vi "DB_LeeIDmedicion.vi"(8 "error in (no error)":errorcluster, 10 "Equipo_Medicion in":T1={"ID_EQUIPO"=0, "IP_EQUIPO"="", "NOMBRE_EQUIPO"="", "ESTADO_EQUIPO"="", "DESCRIPCION"="", "ID_MEDICION"=0, "ESTADO_MEDICION"="", "TIEMPO_MEDICION"="12-02-2019 18:41"}, 11 "db in":T2) -> (0 "error out":errorcluster, 2 "Equipo_Medicion out":T1={"ID_EQUIPO"=0, "IP_EQUIPO"="", "NOMBRE_EQUIPO"="", "ESTADO_EQUIPO"="", "DESCRIPCION"="", "ID_MEDICION"=0, "ESTADO_MEDICION"="", "TIEMPO_MEDICION"="12-02-2019 18:41"}, 3 "db out":T2)   [LabVIEW 2018]
uses:
  <vilib>/addons/database/Connection.llb/Conn ObjectReference.ctl
  Controls/Equipos_Medicion_cluster.ctl
  <vilib>/addons/database/Connection.llb/Conn Execute.vi
  <vilib>/addons/database/Recordset.llb/Rec Fetch Integer Data (R).vi
  <vilib>/addons/database/Recordset.llb/Rec Destroy - Connection.vi
  <vilib>/addons/database/NI_Database_API.lvlib
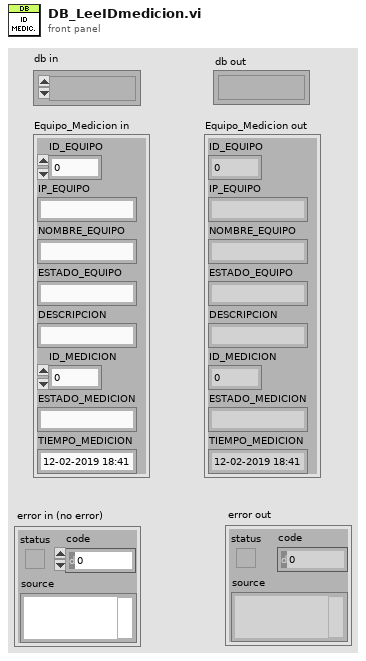
[diagram p1: front panel]
types:
  T1 = typedef "Equipos_Medicion_cluster.ctl" = cluster{"ID_EQUIPO":i32, "IP_EQUIPO":string, "NOMBRE_EQUIPO":string, "ESTADO_EQUIPO":string, "DESCRIPCION":string, "ID_MEDICION":i32, "ESTADO_MEDICION":string, "TIEMPO_MEDICION":string}
  T2 = typedef "NI_Database_API.lvlib/Conn ObjectReference.ctl" = refnum<k1>
  T3 = typedef "NI_Database_API.lvlib/Rec ObjectReference.ctl" = refnum<k1>
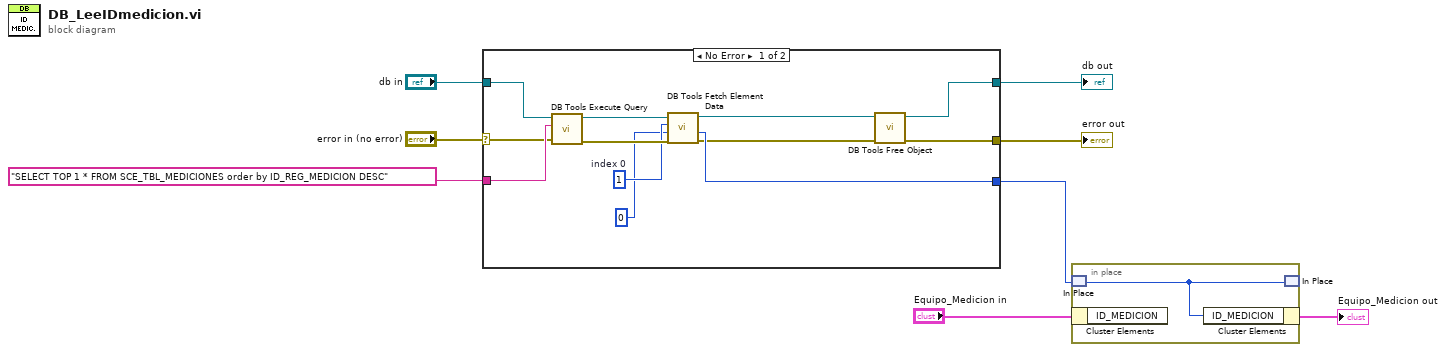
[diagram p0: block diagram]
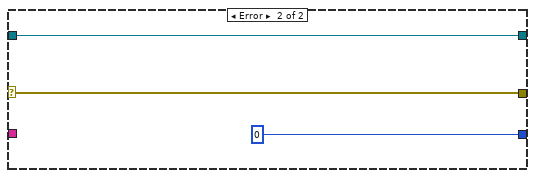
[diagram p2: hidden frame]
diagram:
  n1 = case shown="No Error" "error in (no error)" {
    selector: "error in (no error)" -> [w18 w23]
    tunnel: "SELECT TOP 1 * FROM SCE_TBL_MEDICIONES order by ID_REG_MEDICION DESC" ("SQL") -> [w19 _]
    tunnel: [w17 w23] -> w8
    tunnel: [w14 0] -> w3
    tunnel: "db in" -> [w9 w21]
    tunnel: [w15 w21] -> w4
    frame No Error {
      w13 = 1  # index 0
      n2 = call-poly <vilib>:"DB Tools Execute Query.vi"("error in (no error)"=w18, "SQL query"=w19, "connection reference"=w9) -> ("error out"=w20:errorcluster, "recordset reference"=w10:T3)  [unwired: 5 in]
      n3 = call-poly <vilib>:"DB Tools Fetch Element Data.vi"("error in (no error)"=w20, "type"=0, "column index"=w13, "recordset reference"=w10) -> ("error out"=w11:errorcluster, "data"=w14:i32, "recordset reference out"=w16:T3)  [unwired: 3 in]
      n4 = call-poly <vilib>:"DB Tools Free Object.vi"("error in (no error)"=w11, "recordset reference"=w16) -> ("error out"=w17:errorcluster, "connection reference"=w15:T2)  [unwired: 8 in]
    }
    frame Error {
    }
  }
  "error out" <- w8
  "db out" <- w4
  n5 = in-place {
    n6 = in-place-match #1(w3) -> (w24:i32)
    n7 = in-place-cluster #2("Equipo_Medicion in") -> ()  [unwired: 1 out]
    n8 = in-place-cluster #2("ID_MEDICION"=w24) -> (→"Equipo_Medicion out":T1)
    n9 = in-place-match #1(w24) -> ()  [unwired: 1 out]
  }
